vi "Write To Disk.vi"(8 "error in (no error)":errorcluster, 10 "element":i32[][](array[numeric]), 11 "AcquireTraces in":refnum<class "AcquireTraces.lvclass">) -> (0 "error out":errorcluster, 3 "AcquireTraces out":refnum<class "AcquireTraces.lvclass">)   [LabVIEW 2012, in "AcquisitionCoreObjects.lvlib" / "AcquireTraces.lvclass"]
uses:
  AcquireTraces.lvclass
  AcquireTraces.lvclass/AcquireTraces.ctl
  HDF5Tools/LabView/Append To Dataset 2D Integer.vi
  HDF5Tools/LabView/HDF5Tools.lvlib
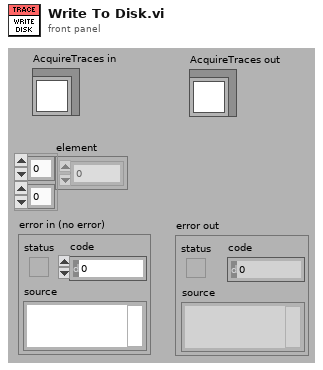
[diagram p1: front panel]
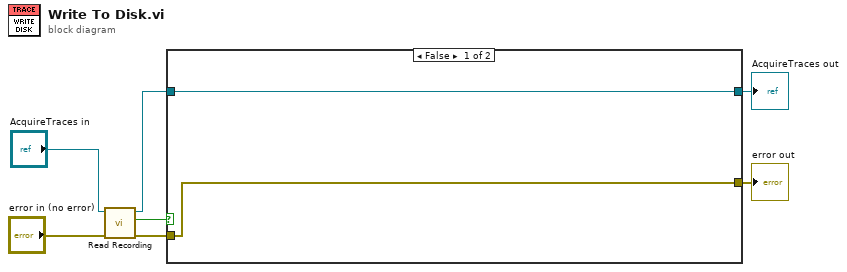
[diagram p0: block diagram]
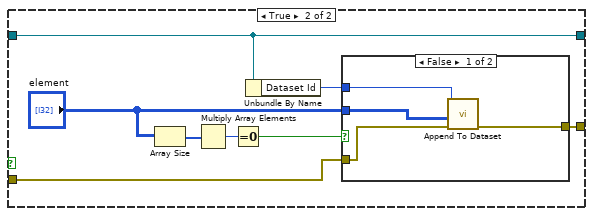
[diagram p2: hidden frame]
diagram:
  n1 = call-dynamic "Read Recording.vi"("error in (no error)"="error in (no error)", "AcquireTraces in"="AcquireTraces in") -> ("error out"=w5:errorcluster, "Recording"=w2:bool, "AcquireTraces out"=w3:refnum<class "AcquireTraces.lvclass">)  [unwired: 7 in]
  n2 = case shown="False" w2 {
    tunnel: w5 -> [w8 w17]
    tunnel: [w8 w16] -> w7
    tunnel: w3 -> [w9 w10]
    tunnel: [w9 w10] -> w1
    frame False {
    }
    frame True {
      n3 = Array Size(array="element") -> (size(s)=w14:i32[])
      n4 = Multiply Array Elements(1:w14) -> (0:w13:i32)
      n5 = Equal To 0?(x=w13) -> (x = 0?=w11:bool)
      n6 = Unbundle By Name(w10) -> ("Dataset Id"=w12:u64)
      n7 = case shown="False" w11 {
        tunnel: "element" -> [w21 _]
        tunnel: w17 -> [w20 _]
        tunnel: [w19 _] -> w16
        tunnel: w12 -> [w18 _]
        frame False {
          n8 = call-poly "Append To Dataset.vi"("error in (no error)"=w20, "data"=w21, "dataset_id"=w18) -> ("error out"=w19:errorcluster)  [unwired: 7 in, 1 out]
        }
        frame True {
        }
      }
    }
  }
  "error out" <- w7
  "AcquireTraces out" <- w1
